vi "ManipEnd.vi"() -> (0 "Error Out":errorcluster, 1 "Advance Trigger":bool)   [LabVIEW 2019]
doc: "Stops the subsystem sequencer.\n\nParameters: None"
uses:
  autoninfo.vi
  dscommands.vi
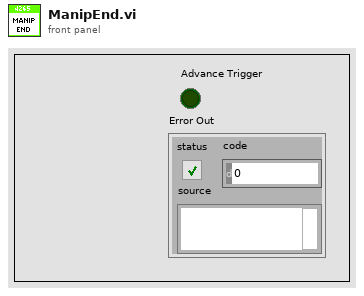
[diagram p1: front panel]
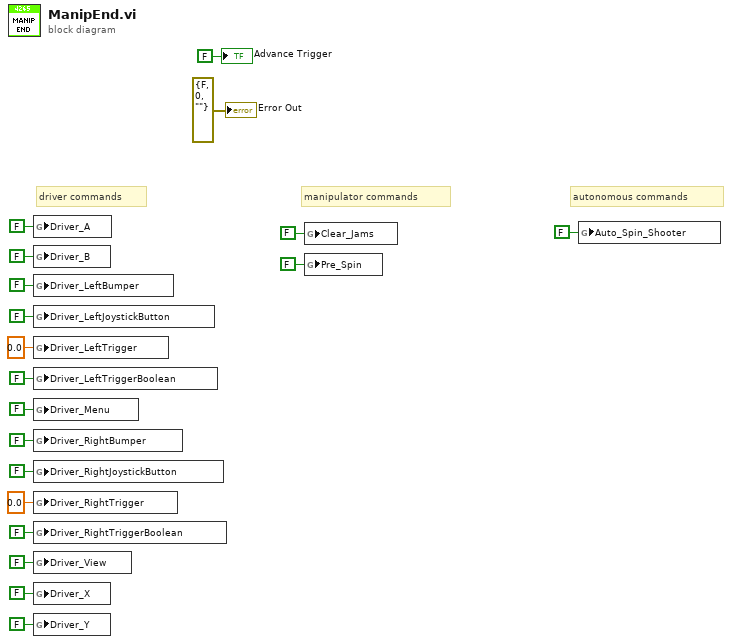
[diagram p0: block diagram]
diagram:
  # "manipulator commands"
  # "driver commands"
  # "autonomous commands"
  n1 = global write "dscommands.vi" "Driver_A"(FALSE ("Driver_A")) -> ()
  n2 = global write "dscommands.vi" "Driver_B"(FALSE ("Driver_B")) -> ()
  n3 = global write "dscommands.vi" "Driver_LeftBumper"(FALSE ("Driver_LeftBumper")) -> ()
  n4 = global write "dscommands.vi" "Driver_LeftJoystickButton"(FALSE ("Driver_LeftJoystickButton")) -> ()
  n5 = global write "dscommands.vi" "Driver_LeftTrigger"(0.0 ("Driver_LeftTrigger")) -> ()
  n6 = global write "dscommands.vi" "Driver_LeftTriggerBoolean"(FALSE ("Driver_LeftTriggerBoolean")) -> ()
  n7 = global write "dscommands.vi" "Driver_Menu"(FALSE ("Driver_Menu")) -> ()
  n8 = global write "dscommands.vi" "Driver_RightBumper"(FALSE ("Driver_RightBumper")) -> ()
  n9 = global write "dscommands.vi" "Driver_RightJoystickButton"(FALSE ("Driver_RightJoystickButton")) -> ()
  n10 = global write "dscommands.vi" "Driver_RightTrigger"(0.0 ("Driver_RightTrigger")) -> ()
  n11 = global write "dscommands.vi" "Driver_RightTriggerBoolean"(FALSE ("Driver_RightTriggerBoolean")) -> ()
  n12 = global write "dscommands.vi" "Driver_View"(FALSE ("Driver_View")) -> ()
  n13 = global write "dscommands.vi" "Driver_X"(FALSE ("Driver_X")) -> ()
  n14 = global write "dscommands.vi" "Driver_Y"(FALSE ("Driver_Y")) -> ()
  n15 = global write "dscommands.vi" "Clear_Jams"(FALSE ("Clear_Jams")) -> ()
  n16 = global write "dscommands.vi" "Pre_Spin"(FALSE ("Clear_Jams")) -> ()
  n17 = global write "autoninfo.vi" "Auto_Spin_Shooter"(FALSE ("Auto_Spin_Shooter")) -> ()
  "Advance Trigger" <- FALSE ("Advance Trigger")
  "Error Out" <- errorcluster {"status"=FALSE, "code"=0, "source"=""} ("error constant")
